vi "Enqueue Item.vi"(8 "error in (no error)":errorcluster, 9 "Message":variant, 10 "State":string, 11 "Queue in":refnum<queue>) -> (0 "error out":errorcluster, 3 "Queue out":refnum<queue>)   [LabVIEW 2016]
uses:
  Type Defs/Message.ctl
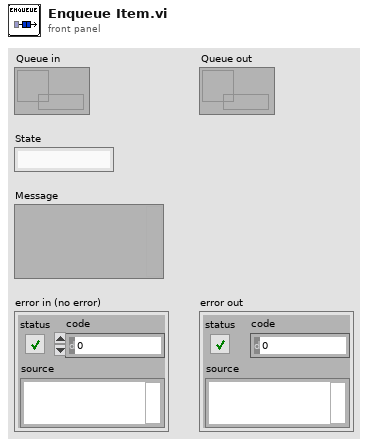
[diagram p1: front panel]
types:
  T1 = typedef "Message.ctl" = cluster{"State":string, "Message":variant}
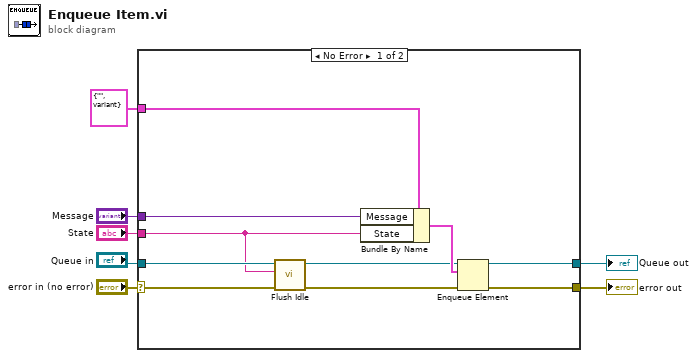
[diagram p0: block diagram]
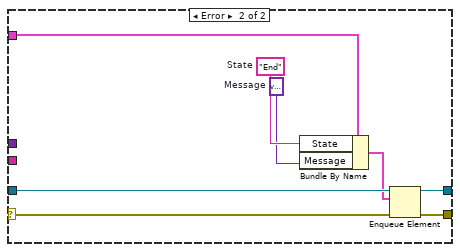
[diagram p2: hidden frame]
diagram:
  n1 = case shown="No Error" "error in (no error)" {
    selector: "error in (no error)" -> [w9 w20]
    tunnel: [w17 w25] -> w7
    tunnel: [w16 w24] -> w6
    tunnel: "Queue in" -> [w12 w23]
    tunnel: T1 {"State"="", "Message"=variant} ("Cluster") -> [w15 w22]
    tunnel: "State" -> [w8 _]
    tunnel: "Message" -> [w13 _]
    frame No Error {
      n2 = call "Flush Idle.vi"("error in (no error)"=w9, "State"=w8, "Queue in"=w12) -> ("error out"=w10:errorcluster, "Queue out"=w11:refnum<queue>)  [unwired: 7 in]
      n3 = Bundle By Name(cluster=w15, "Message"=w13, "State"=w8) -> (w14:T1)
      n4 = Enqueue Element(queue=w11, element=w14, error in (no error)=w10) -> (queue out=w16:refnum<queue>, error out=w17:errorcluster)  [unwired: 1 in, 1 out]
    }
    frame Error {
      w18 = variant  # Message
      w19 = "End"  # State
      n5 = Bundle By Name(cluster=w22, "State"=w19, "Message"=w18) -> (w21:T1)
      n6 = Enqueue Element(queue=w23, element=w21, error in (no error)=w20) -> (queue out=w24:refnum<queue>, error out=w25:errorcluster)  [unwired: 1 in, 1 out]
    }
  }
  "error out" <- w7
  "Queue out" <- w6
